vi "ValidateResults2.vi"(9 "PowerSpectrum2 (in)":sgl[](array[numeric]), 10 "PowerSpectrum1 (in)":sgl[](array[numeric]), 11 "Max Error":sgl=0.001) -> (2 "Errors":cluster{"lower limit":sgl, "Index":i32}[](array[cluster]), 3 "Results Match?":bool)   [LabVIEW 2015, in "SETI_LV.lvlib"]
uses:
  SETI_LV.lvlib
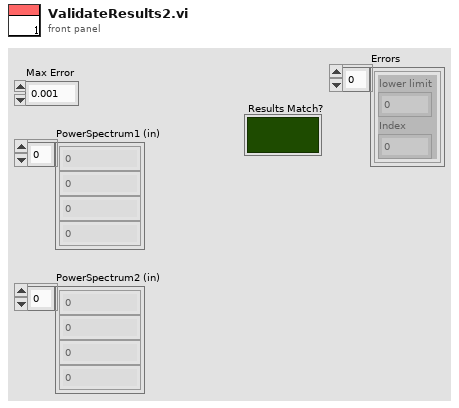
[diagram p1: front panel]
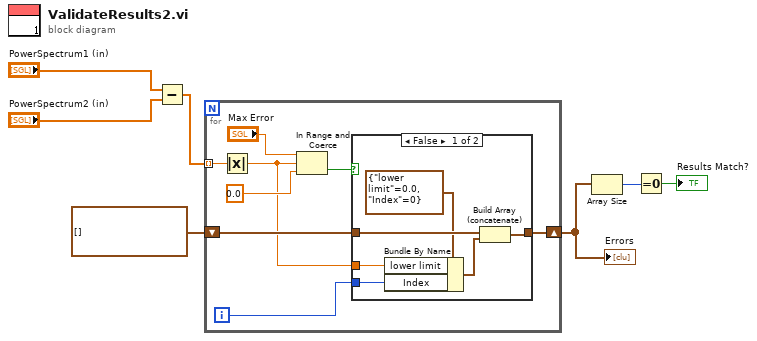
[diagram p0: block diagram]
diagram:
  n1 = Subtract(x="PowerSpectrum1 (in)", y="PowerSpectrum2 (in)") -> (x-y=w5:sgl[])
  n2 = for {
    tunnel: w5 -> [w9] mode=indexing
    shift-right: [w11] -> w3
    shift-left: cluster{"lower limit":sgl, "Index":i32}[] [] -> [w12]
    i -> [w10]
    n3 = Absolute Value(x=w9) -> (abs(x)=w8:sgl)
    n4 = In Range and Coerce(upper limit="Max Error", x=w8, lower limit=sgl 0.0) -> (In Range?=w13:bool)  [unwired: 1 out]
    n5 = case shown="False" w13 {
      tunnel: w12 -> [w20 w22]
      tunnel: [w21 w22] -> w11
      tunnel: w10 -> [w18 _]
      tunnel: w8 -> [w17 _]
      frame False {
        n6 = Bundle By Name(cluster=cluster{"lower limit":sgl, "Index":i32} {"lower limit"=0.0, "Index"=0} ("Cluster"), "lower limit"=w17, "Index"=w18) -> (w19:cluster{"lower limit":sgl, "Index":i32})
        n7 = Build Array (concatenate)(w20, w19) -> (w21:cluster{"lower limit":sgl, "Index":i32}[])
      }
      frame True {
      }
    }
  }
  "Errors" <- w3
  n8 = Array Size(array=w3) -> (size(s)=w2:i32)
  n9 = Equal To 0?(x=w2) -> (x = 0?=→"Results Match?":bool)
